vi "AUTO_HOME.vi"(8 "error in (no error)":errorcluster) -> (0 "error out":errorcluster)   [LabVIEW 2017]
doc: "This vi is for manually turn ON and OFF also monitor Output of PLCS. So this is manual screen."
uses:
  b56ad881-f772-481a-9ad8-33fdffb2c092.vi
  Global/PLC_to_Auto.vi
  <vilib>/Utility/file.llb/Read Delimited Spreadsheet (string).vi
  <vilib>/Utility/file.llb/Write Delimited Spreadsheet (string).vi
panel:
  out "AUTO\nHOME STOP":bool
  in  "SPRING ABORT":bool
  in  "SPRING ACK":bool
  out "PART OK":bool
  out "SYSTEM READY":bool
  out "HAUSING STATUS":bool
  out "MAGNETIC STATUS":bool
  out "CBCT STATUS":bool
  out "PMR STATUS":bool
  out "KINEMATIC STATUS":bool
  out "KITTING ST NG COUNTER":u16 format="NG COUNTER: %.0f"
  out "KITTING ST OK COUNTER":u16 format="OK COUNTER: %.0f"
  out "KITTING ST CYCLE TIME":dbl format="CYCLE TIME : %.1f SEC"
  out "CYCLE STATUS 10":bool
  out "CYCLE STATUS 8":bool
  out "CYCLE STATUS 4":bool
  out "CYCLE STATUS 7":bool
  out "CYCLE STATUS 3":bool
  out "CYCLE STATUS 6":bool
  out "CYCLE STATUS 2":bool
  out "CYCLE STATUS 5":bool
  out "CYCLE STATUS 1":bool
  out "CYCLE TIME IN SEC":T1 {"CYCLE TIME 10" format="%.1f"; "CYCLE TIME 8" format="%.1f"; "CYCLE TIME 4" format="%.1f"; "CYCLE TIME 7" format="%.1f"; "CYCLE TIME 3" format="%.1f"; "CYCLE TIME 6" format="%.1f"; "CYCLE TIME 2" format="%.1f"; "CYCLE TIME 5" format="%.1f"; "CYCLE TIME 1" format="%.1f"}
  out "BOOLEAN 2":bool
  out "Plan Selected:":string
  out "USER:-":string
  out "ALARM Indicator":string
  out "DATE/TIME":string
  in  "Back":bool
  # "AUTO HOME"
  # "7.NEUTRAL\n2B ASSEMBLY"
  # "4.NEUTRAL\nIA ASSEMBLY"
  # "6.NEUTRAL\n2A ASSEMBLY"
  # "5.NEUTRAL\nIB ASSEMBLY"
  # "3.PHASE SIDE\nII ASSEMBLY"
  # "10.FINAL\nVISION SYSTEM"
  # "8.NEUTRAL\n2C ASSEMBLY"
  # "2.PHASE SIDE\nI ASSEMBLY"
  # "1.KITTING \nSTATION"
  # "CYCLE TIME IN SEC"
  # "OK COUNTER"
  # "NG COUNTER"
  # "CYCLE STATUS"
  # "ALARM:-"
  # "STATUS OF\n KITTING STATION"
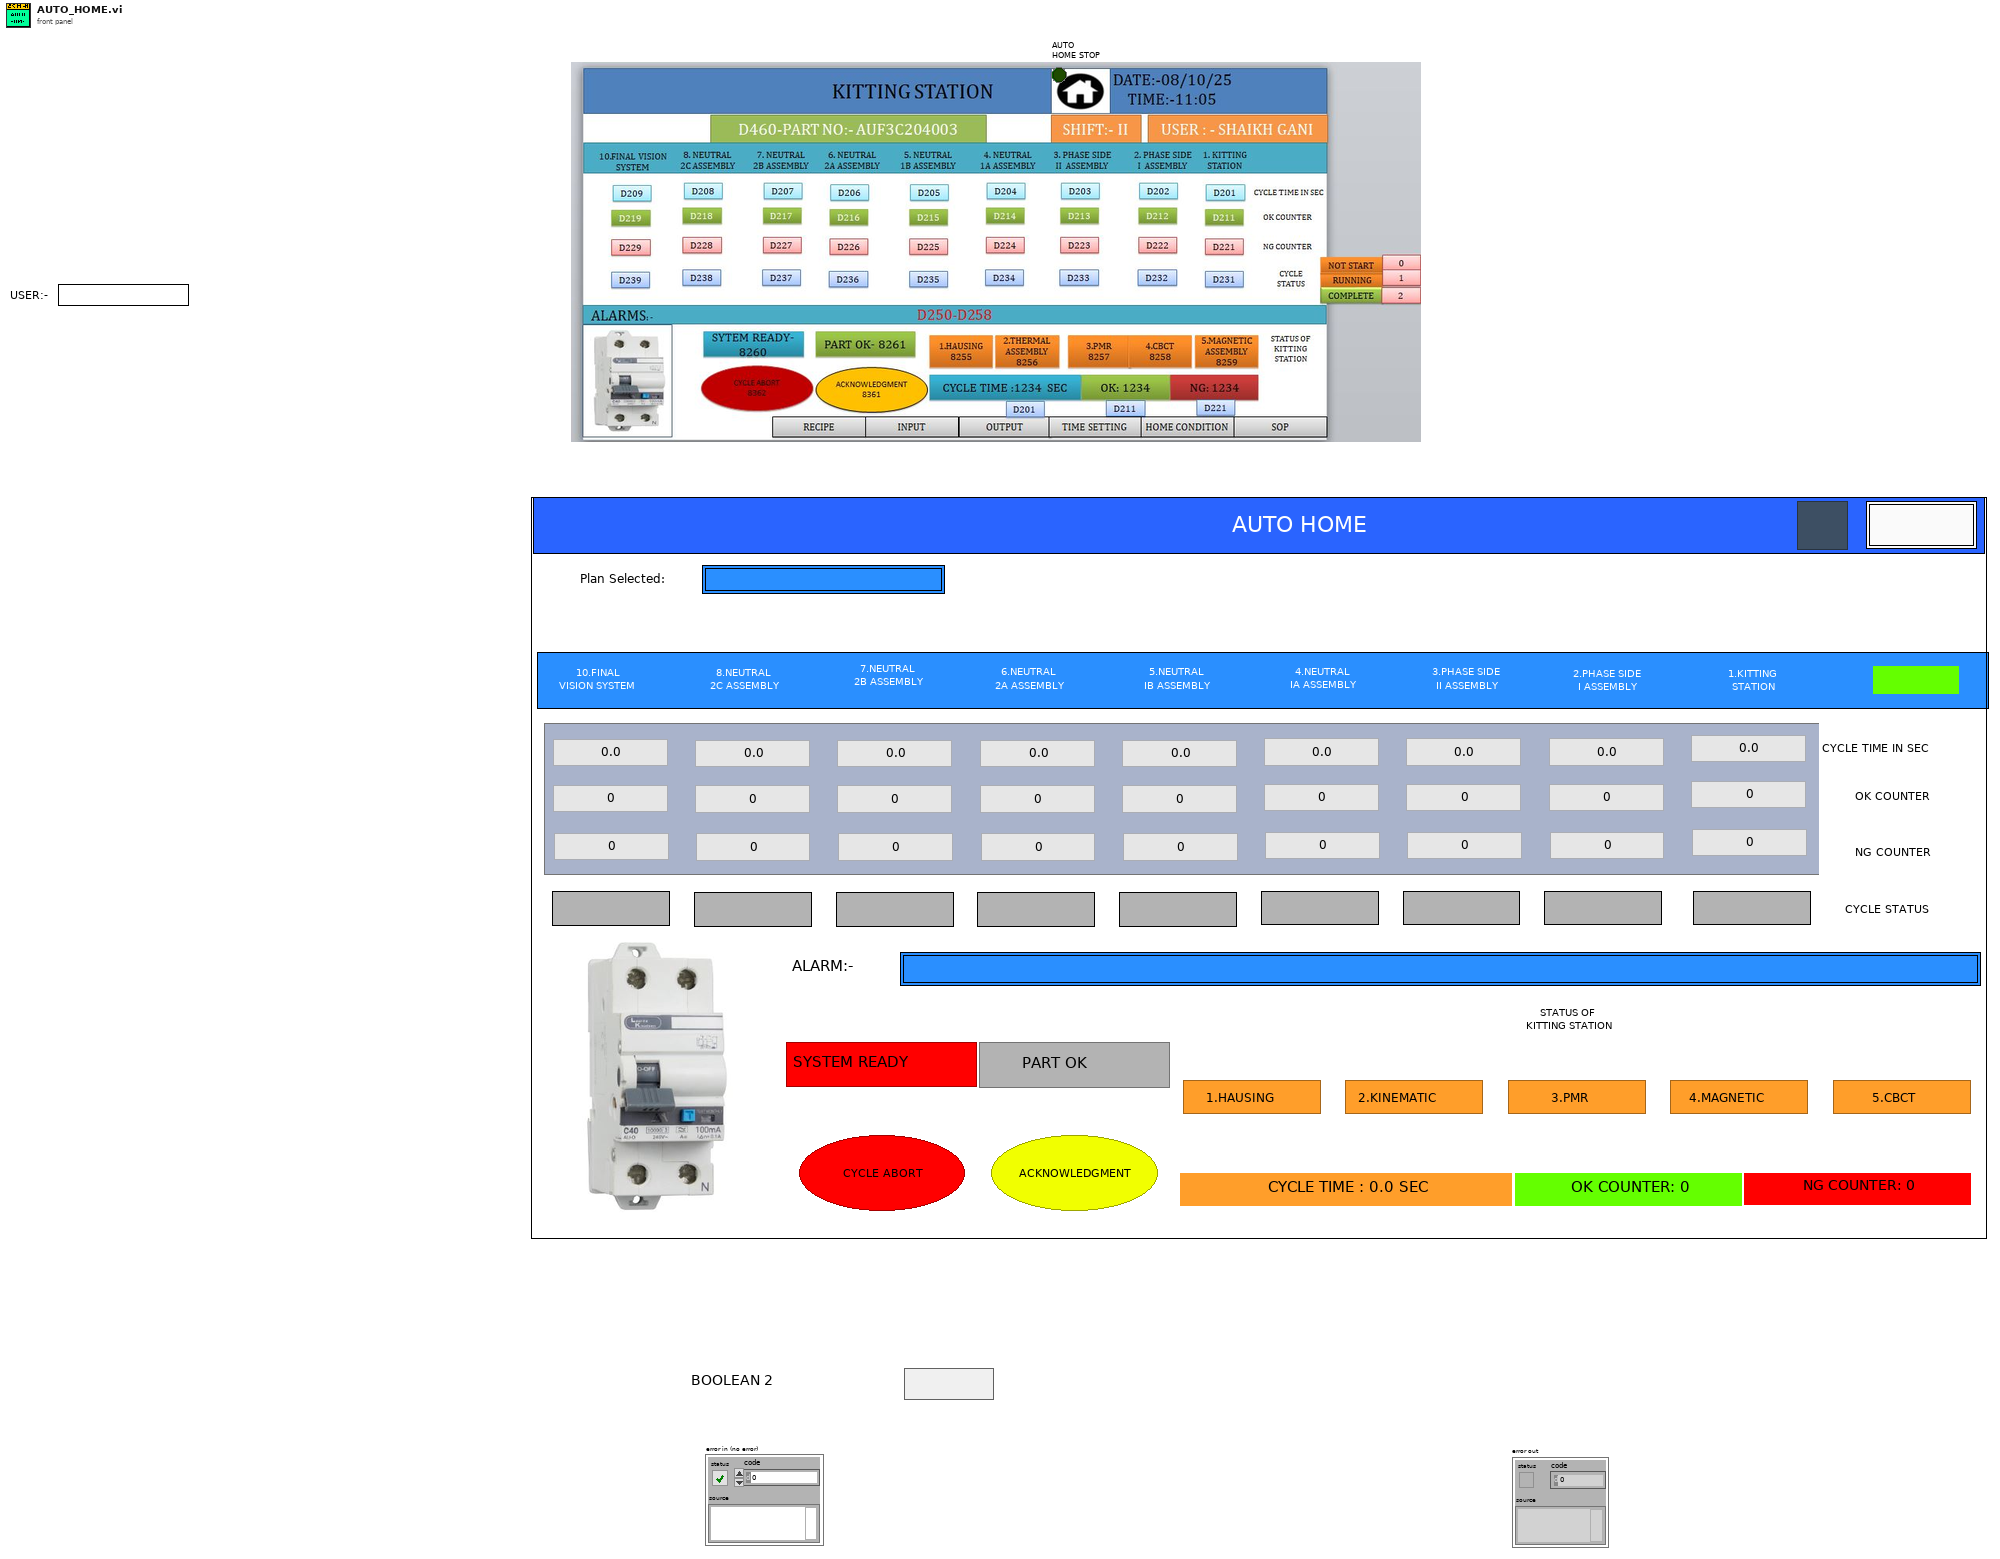
[diagram p1: front panel]
types:
  T1 = cluster{"CYCLE TIME 1":dbl, "CYCLE TIME 2":dbl, "CYCLE TIME 3":dbl, "CYCLE TIME 4":dbl, "CYCLE TIME 5":dbl, "CYCLE TIME 6":dbl, "CYCLE TIME 7":dbl, "CYCLE TIME 8":dbl, "CYCLE TIME 10":dbl, "CYCLE TIME 9":u16, "CYCLE TIME 12":u16, "CYCLE TIME 14":u16, "CYCLE TIME 16":u16, "CYCLE TIME 11":u16, "CYCLE TIME 13":u16, "CYCLE TIME 15":u16, "CYCLE TIME 17":u16, "CYCLE TIME 18":u16, "CYCLE TIME 19":u16, "CYCLE TIME 21":u16, "CYCLE TIME 23":u16, "CYCLE TIME 25":u16, "CYCLE TIME 20":u16, "CYCLE TIME 22":u16, "CYCLE TIME 24":u16, "CYCLE TIME 26":u16, "CYCLE TIME 27":u16}
  T2 = enum32{"invalid app kind", "Development System", "Run Time System", "Student Edition", "Embedded LabVIEW", "Evaluation", "Custom"}
  T3 = cluster{"[0]":dbl, "[1]":dbl, "[2]":dbl, "[3]":dbl, "[4]":dbl, "[5]":dbl, "[6]":dbl, "[7]":dbl, "[8]":dbl, "[9]":dbl, "[10]":dbl, "[11]":dbl, "[12]":dbl, "[13]":dbl, "[14]":dbl, "[15]":dbl, "[16]":dbl, "[17]":dbl, "[18]":dbl, "[19]":dbl, "[20]":dbl, "[21]":dbl, "[22]":dbl, "[23]":dbl, "[24]":dbl, "[25]":dbl, "[26]":dbl}
  T4 = enum32{"Invalid", "Standard", "Closed", "Hidden", "Minimized", "Maximized"}
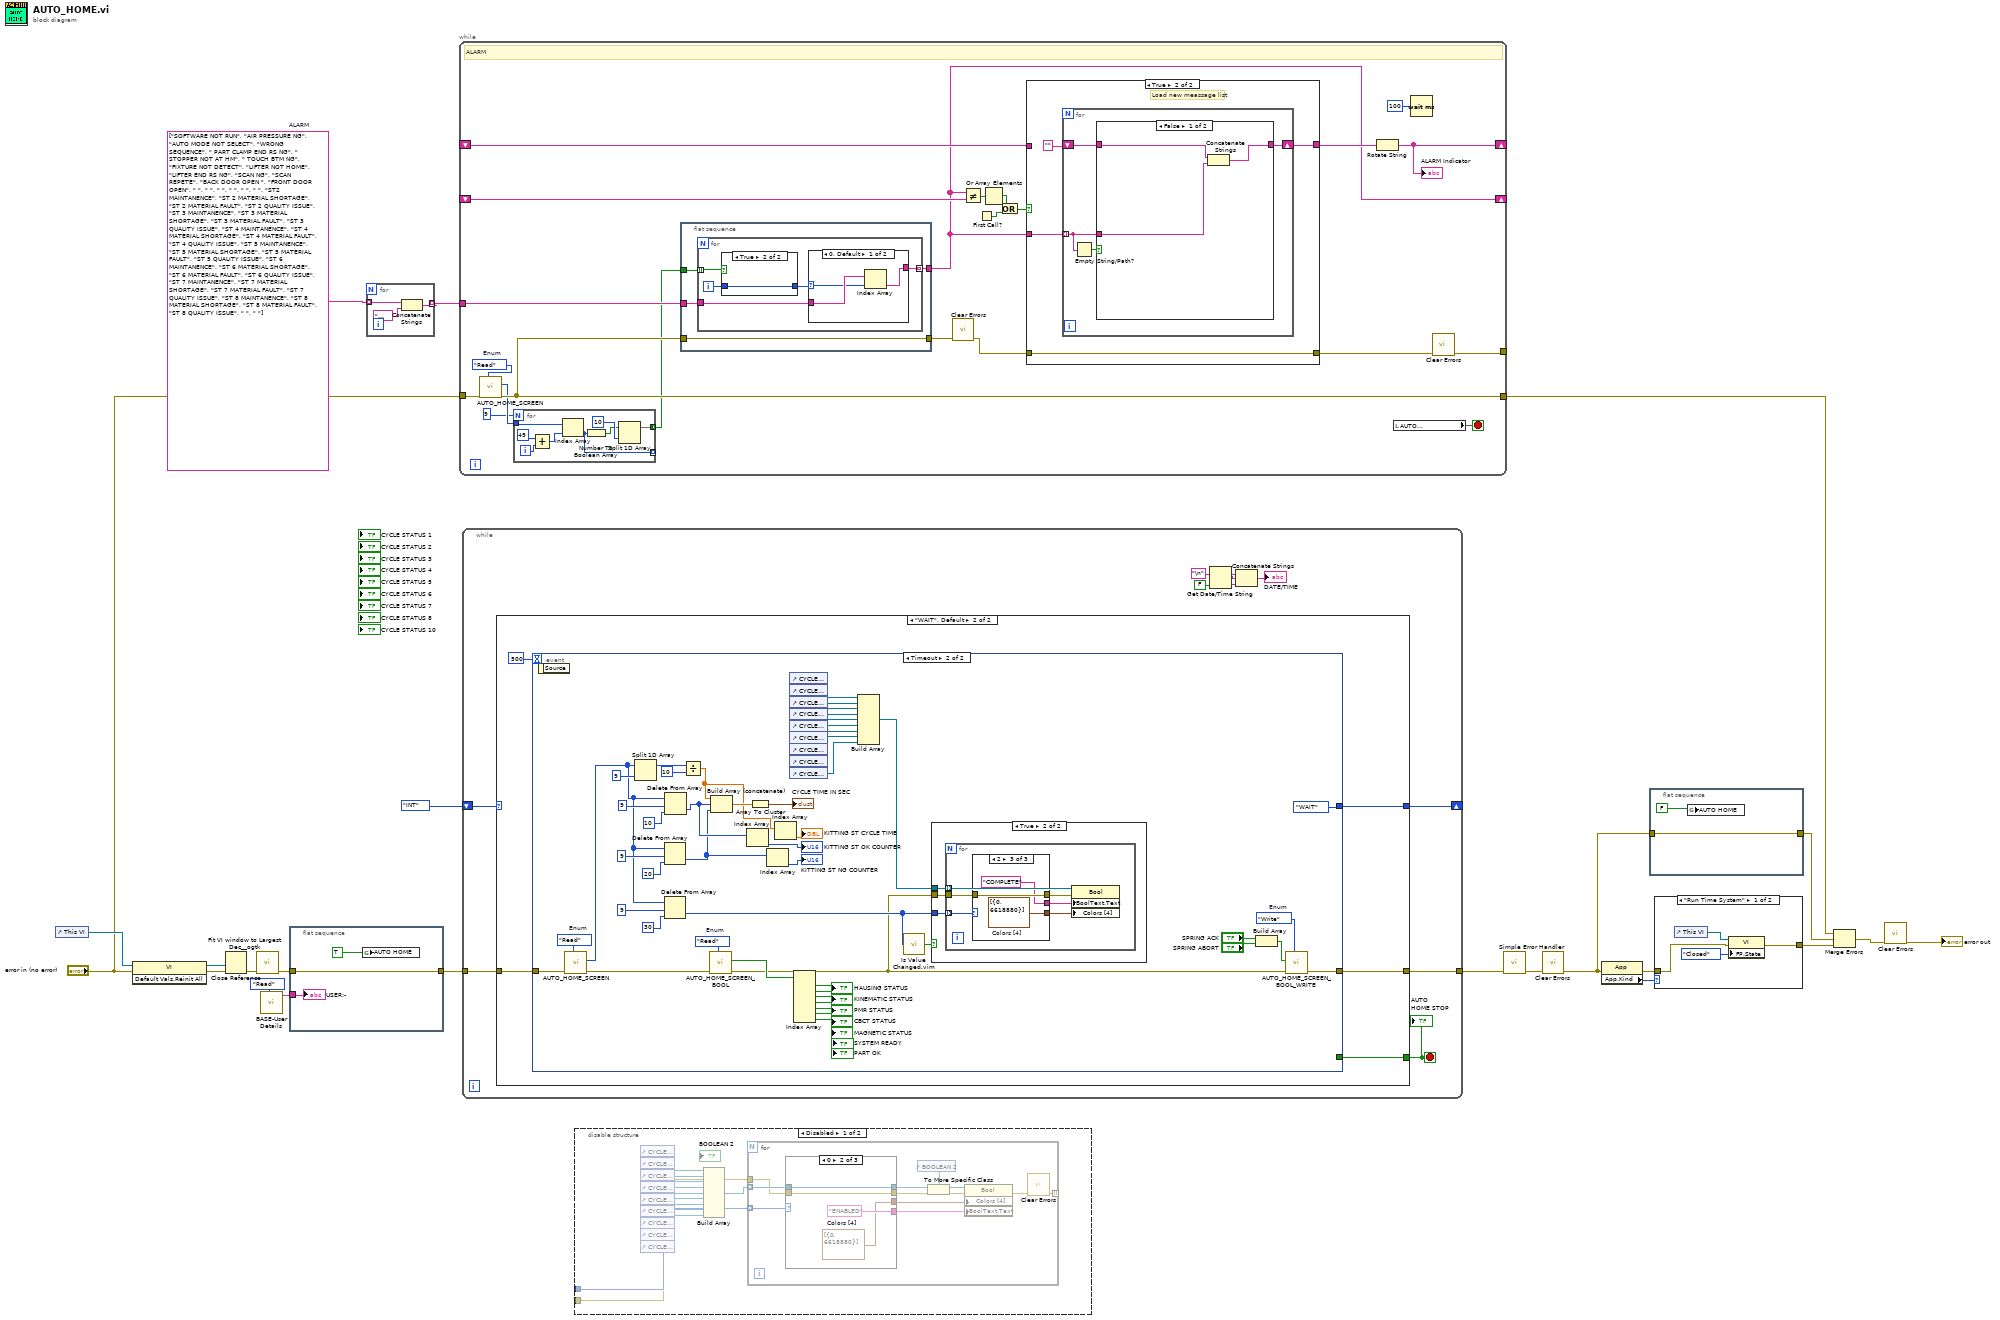
[diagram p0: block diagram]
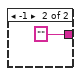
[diagram p2: hidden frame]
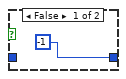
[diagram p3: hidden frame]
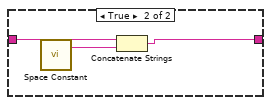
[diagram p5: hidden frame]
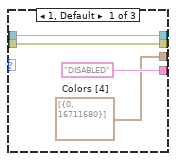
[diagram p6: hidden frame]
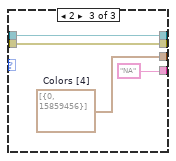
[diagram p7: hidden frame]
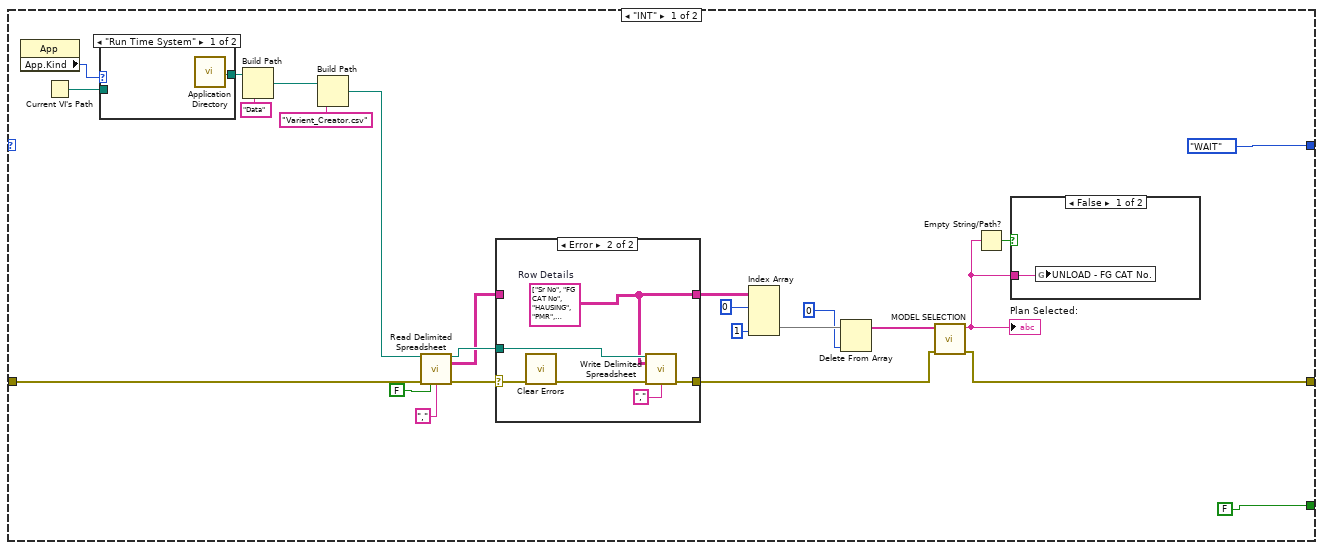
[diagram p10: hidden frame]
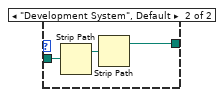
[diagram p12: hidden frame]
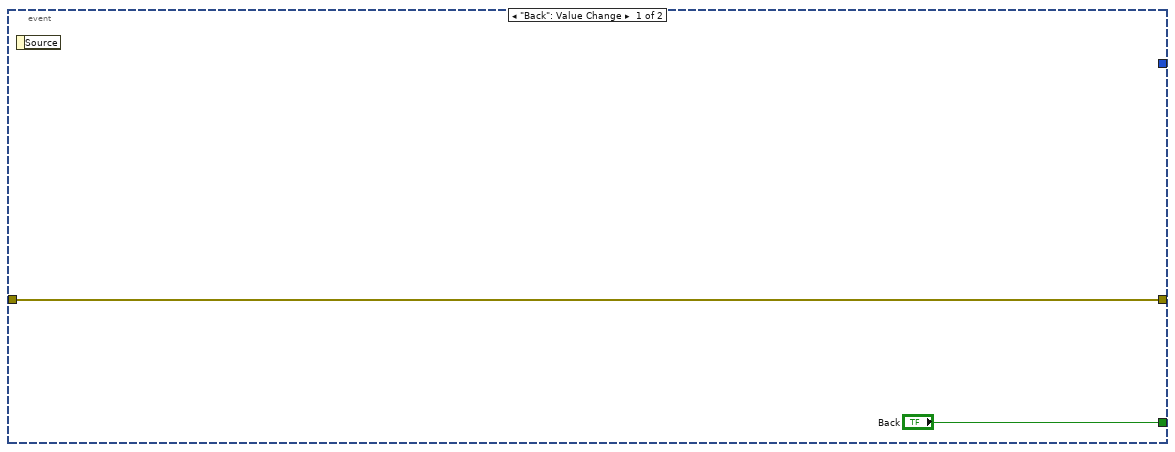
[diagram p14: hidden frame]
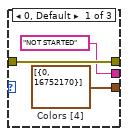
[diagram p16: hidden frame]
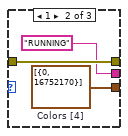
[diagram p17: hidden frame]
diagram:
  w1 = string[] ["SOFTWARE NOT RUN", "AIR PRESSURE NG", "AUTO MODE NOT SELECT", "WRONG SEQUENCE", " PART CLAMP END RS NG", " STOPPER NOT AT HM", " TOUCH BTM NG", "FIXTURE NOT DETECT", "LIFTER NOT HOME", "LIFTER END RS NG", "SCAN NG", "SCAN  REPETE", "BACK DOOR OPEN ", "FRONT DOOR OPEN", " ", " ", " ", " ", " ", " ", "ST2 MAINTANENCE", "ST 2 MATERIAL SHORTAGE", "ST 2 MATERIAL FAULT", "ST 2 QUALITY ISSUE", "ST 3 MAINTANENCE", "ST 3 MATERIAL SHORTAGE", "ST 3 MATERIAL FAULT", "ST 3 QUALITY ISSUE", "ST 4 MAINTANENCE", "ST 4 MATERIAL SHORTAGE", "ST 4 MATERIAL FAULT", "ST 4 QUALITY ISSUE", "ST 5 MAINTANENCE", "ST 5 MATERIAL SHORTAGE", "ST 5 MATERIAL FAULT", "ST 5 QUALITY ISSUE", "ST 6 MAINTANENCE", "ST 6 MATERIAL SHORTAGE", "ST 6 MATERIAL FAULT", "ST 6 QUALITY ISSUE", "ST 7 MAINTANENCE", "ST 7 MATERIAL SHORTAGE", "ST 7 MATERIAL FAULT", "ST 7 QUALITY ISSUE", "ST 8 MAINTANENCE", "ST 8 MATERIAL SHORTAGE", "ST 8 MATERIAL FAULT", "ST 8 QUALITY ISSUE", " ", " "]  # ALARM
  n1 = control-ref of="This VI"() -> (w18:refnum<vi>)
  n2 = invoke class="VI" method="Default Vals.Reinit All"(reference=w18, error in="error in (no error)") -> (reference out=w17:refnum<vi>, error out=w16:errorcluster)  [unwired: 1 in, 1 out]
  n3 = Close Reference(reference=w17, error in (no error)=w16) -> (error out=w15:errorcluster)
  n4 = call <userlib>:"Fit VI window to Largest Dec__ogtk.vi"("error in (no error)"=w15) -> ("error out"=w14:errorcluster)  [unwired: 5 in, 1 out]
  n5 = call "BASE-User Details.vi"("Enum"=enum16{"Read", "Write"}."Read") -> ("User Name Out"=w6:string)  [unwired: 9 in, 1 out]
  n6 = flat-sequence {
    tunnel: w14 -> [w25]
    tunnel: [w25] -> w10
    tunnel: w6 -> [w23]
    frame #0 {
      n7 = global write "PLC_to_Auto.vi" "AUTO HOME"(TRUE) -> ()
      "USER:-" <- w23
    }
  }
  n8 = for {
    tunnel: w1 -> [w28] mode=indexing
    tunnel: [w26] -> w4 mode=indexing
    n9 = Concatenate Strings(w28, "          ") -> (w26:string)
  }
  n10 = while {
    tunnel: "error in (no error)" -> [w34]
    tunnel: [w39] -> _
    tunnel: w4 -> [w37]
    shift-right: [w35] -> _
    shift-left: _ -> [w46]
    shift-right: [w45] -> _
    shift-left: _ -> [w47]
    tunnel: [w33] -> w2
    stop <- w36 stop-if-true
    w32 = enum16{"Read", "Write"}."Read"  # Enum
    # "ALARM"
    n11 = call "AUTO_HOME_SCREEN.vi"("Enum"=w32, "error in (no error)"=w34) -> ("error out"=w33:errorcluster, "Array 2"=w31:u16[])  [unwired: 8 in]
    n12 = for {
      N: 9 -> [_]
      tunnel: w31 -> [w58]
      tunnel: [w52] -> w29 mode=concatenating
      tunnel: [w51] -> _ mode=indexing
      i -> [w56]
      n13 = Add(x=49, y=w56) -> (x+y=w55:i32)
      n14 = Index Array(array=w58, index=w55) -> (element=w51:u16)
      n15 = Number To Boolean Array(number=w51) -> (Boolean array=w53:bool[])
      n16 = Split 1D Array(array=w53, index=10) -> (first subarray=w52:bool[])  [unwired: 1 out]
    }
    n17 = flat-sequence {
      tunnel: [w60] -> w41
      tunnel: [w62] -> w45
      tunnel: w37 -> [w61]
      tunnel: w33 -> [w60]
      tunnel: w29 -> [w59]
      frame #0 {
        n18 = for {
          tunnel: w59 -> [w67] mode=indexing
          tunnel: [w63] -> w62 mode=indexing
          tunnel: w61 -> [w65]
          i -> [w66]
          n19 = case shown="True" w67 {
            tunnel: w66 -> [_ w73]
            tunnel: [-1 w73] -> w64
            frame False {
            }
            frame True {
            }
          }
          n20 = case shown="0, Default" w64 {
            selector: w64 -> [w69 _]
            tunnel: w65 -> [w70 _]
            tunnel: [w68 ""] -> w63
            frame 0, Default {
              n21 = Index Array(array=w70, index=w69) -> (element=w68:string)
            }
            frame -1 {
            }
          }
        }
      }
    }
    n22 = call <vilib>:"Clear Errors.vi"("error in (no error)"=w41) -> ("error out"=w40:errorcluster)  [unwired: 5 in, 1 out]
    n23 = Not Equal?(x=w45, y=w47) -> (x != y?=w49:bool[])
    n24 = First Call?() -> (First Call?: T/F=w44:bool)
    n25 = Or Array Elements(Boolean array=w49) -> (logical OR=w43:bool)
    n26 = Or(x=w43, y=w44) -> (x .or. y?=w42:bool)
    n27 = case shown="True" w42 {
      tunnel: [w75 w77] -> w48
      tunnel: w46 -> [w75 _]
      tunnel: w45 -> [_ w78]
      tunnel: w40 -> [w74 w76]
      tunnel: [w74 w76] -> w38
      frame False {
      }
      frame True {
        # "Load new meassage list"
        n28 = for {
          tunnel: w78 -> [w81] mode=indexing
          shift-right: [w83] -> w77
          shift-left: "" -> [w82]
          n29 = Empty String/Path?(string/path=w81) -> (empty?=w80:bool)
          n30 = case shown="False" w80 {
            tunnel: [w86 w89] -> w83
            tunnel: w82 -> [w85 w88]
            tunnel: w81 -> [w84 _]
            frame False {
              n31 = Concatenate Strings(w85, w84) -> (w86:string)
            }
            frame True {
              n32 = call <vilib>:"Space Constant.vi"() -> ("String"=w87:string)
              n33 = Concatenate Strings(w88, w87) -> (w89:string)
            }
          }
        }
      }
    }
    n34 = Rotate String(1:w48) -> (0:w35:string)
    "ALARM Indicator" <- w35
    n35 = local read "AUTO\nHOME STOP"() -> (w36:bool)
    n36 = Wait (ms)(milliseconds to wait=u32 100) -> ()  [unwired: 1 out]
    n37 = call <vilib>:"Clear Errors.vi"("error in (no error)"=w38) -> ("error out"=w39:errorcluster)  [unwired: 5 in, 1 out]
  }
  n38 = while {
    tunnel: w10 -> [w99]
    tunnel: [w98] -> w21
    shift-right: [w95] -> _
    shift-left: enum16{"INT", "WAIT"}."INT" -> [w96]
    stop <- w97 stop-if-true
    n39 = case shown="\"WAIT\", Default" w96 {
      tunnel: w99 -> [w116 w142]
      tunnel: [w106 w141] -> w98
      tunnel: [FALSE w140] -> w97
      tunnel: [enum16{"INT", "WAIT"}."WAIT" w138] -> w95
      frame "INT" {
        n40 = property class="App"() -> ("App.Kind"=w114:T2)  [unwired: 2 in, 2 out]
        n41 = Current VI's Path() -> (path=w115:path)
        n42 = case shown="\"Run Time System\"" w114 {
          tunnel: w115 -> [_ w128]
          tunnel: [w126 w127] -> w112
          frame "Run Time System" {
            n43 = call <vilib>:"Application Directory.vi"() -> ("Application Directory"=w126:path)
          }
          frame "Development System", Default {
            n44 = Strip Path(path=w128) -> (stripped path=w129:path)  [unwired: 1 out]
            n45 = Strip Path(path=w129) -> (stripped path=w127:path)  [unwired: 1 out]
          }
        }
        n46 = Build Path(base path=w112, name or relative path="Data") -> (appended path=w110:path)
        n47 = Build Path(base path=w110, name or relative path="Varient_Creator.csv") -> (appended path=w109:path)
        n48 = call-poly <vilib>:"Read Delimited Spreadsheet.vi"("file path (dialog if empty)"=w109, "error in (no error)"=w116, "transpose? (F)"=FALSE, "delimiter (\\t)"=",") -> ("new file path (Not A Path if cancelled)"=w121:path, "all rows"=w120:string[][], "error out"=w122:errorcluster)  [unwired: 6 in, 3 out]
        n49 = case shown="Error" w122 {
          selector: w122 -> [w131 w137]
          tunnel: [w131 w135] -> w108
          tunnel: w121 -> [_ w134]
          tunnel: [w130 w132] -> w117
          tunnel: w120 -> [w130 _]
          frame No Error {
          }
          frame Error {
            w132 = string[][] [["Sr No", "FG CAT No", "HAUSING", "PMR", "MAGNETIC ASLY", "CBCT GROUP", "KINEMATIC ASLY", "TEST RESISTOR"]]  # Row Details
            n50 = call <vilib>:"Clear Errors.vi"("error in (no error)"=w137) -> ("error out"=w136:errorcluster)  [unwired: 5 in, 1 out]
            n51 = call-poly <vilib>:"Write Delimited Spreadsheet.vi"("file path (dialog if empty)"=w134, "2D data"=w132, "error in (no error)"=w136, "delimiter (\\t)"=",") -> ("error out"=w135:errorcluster)  [unwired: 10 in, 1 out]
          }
        }
        n52 = Index Array(array=w117, index (row) #1=0, index (col) #2=1) -> (element #2=w104:string[])  [unwired: 2 in, 1 out]
        n53 = Delete From Array(array=w104, index=0) -> (array with subset deleted=w103:string[])  [unwired: 1 in, 1 out]
        n54 = call "MODEL SELECTION.vi"("error in (no error)"=w108, "Plan List"=w103) -> ("error out 2"=w106:errorcluster, "Plan Selected"=w100:string)  [unwired: 7 in, 1 out]
        "Plan Selected:" <- w100
        n55 = Empty String/Path?(string/path=w100) -> (empty?=w101:bool)
        n56 = case shown="False" w101 {
          tunnel: w100 -> [w125 _]
          frame False {
            n57 = global write "PLC_to_Auto.vi" "UNLOAD - FG CAT No."(w125) -> ()
          }
          frame True {
          }
        }
      }
      frame "WAIT", Default {
        n58 = event shown="[1] Timeout" {
          selector: _ -> [_ _]
          dyn-events: _ -> [_ _]
          timeout: 500 -> [_ _]
          tunnel: w142 -> [w143 w191]
          tunnel: [w143 w146] -> w141
          tunnel: ["Back" _] -> w140
          tunnel: [_ enum16{"INT", "WAIT"}."WAIT"] -> w138
          event "Back": Value Change {
            n59 = event-data() -> ()  [unwired: 1 in, 1 out]
          }
          event Timeout {
            w145 = enum16{"Read", "Write"}."Write"  # Enum
            w151 = enum16{"Read", "Write"}."Read"  # Enum
            w192 = enum16{"Read", "Write"}."Read"  # Enum
            n60 = event-data() -> ()  [unwired: 1 in, 1 out]
            n61 = call "AUTO_HOME_SCREEN.vi"("Enum"=w192, "error in (no error)"=w191) -> ("error out"=w152:errorcluster, "Array 2"=w179:u16[])  [unwired: 8 in]
            n62 = Split 1D Array(array=w179, index=9) -> (first subarray=w183:u16[])  [unwired: 1 out]
            n63 = Delete From Array(array=w179, length=9 ("index"), index=20) -> (deleted portion=w161:u16[])  [unwired: 1 out]
            n64 = Delete From Array(array=w179, length=9 ("index"), index=30) -> (deleted portion=w167:u16[])  [unwired: 1 out]
            n65 = Delete From Array(array=w179, length=9 ("index"), index=10) -> (deleted portion=w162:u16[])  [unwired: 1 out]
            n66 = Divide(x=w183, y=10 ("index")) -> (x/y=w163:dbl[])
            n67 = call "AUTO_HOME_SCREEN_BOOL.vi"("Enum"=w151, "error in (no error)"=w152) -> ("error out"=w147:errorcluster, "Array 2"=w153:bool[])  [unwired: 8 in]
            n68 = Build Array (concatenate)(w163, w162, w161) -> (w186:dbl[])
            n69 = Index Array(array=w162) -> (element=→"KITTING ST OK COUNTER":u16)  [unwired: 1 in]
            n70 = Array To Cluster(array=w186) -> (cluster=→"CYCLE TIME IN SEC":T3)
            n71 = Index Array(array=w161) -> (element=→"KITTING ST NG COUNTER":u16)  [unwired: 1 in]
            n72 = Index Array(array=w163) -> (element=→"KITTING ST CYCLE TIME":dbl)  [unwired: 1 in]
            n73 = control-ref of="CYCLE STATUS 1"() -> (w178:refnum<vi>)
            n74 = control-ref of="CYCLE STATUS 2"() -> (w177:refnum<vi>)
            n75 = control-ref of="CYCLE STATUS 3"() -> (w176:refnum<vi>)
            n76 = control-ref of="CYCLE STATUS 4"() -> (w175:refnum<vi>)
            n77 = control-ref of="CYCLE STATUS 5"() -> (w174:refnum<vi>)
            n78 = control-ref of="CYCLE STATUS 6"() -> (w173:refnum<vi>)
            n79 = control-ref of="CYCLE STATUS 7"() -> (w172:refnum<vi>)
            n80 = control-ref of="CYCLE STATUS 8"() -> (w171:refnum<vi>)
            n81 = control-ref of="CYCLE STATUS 10"() -> (w170:refnum<vi>)
            n82 = Index Array(array=w153) -> (element #1=→"HAUSING STATUS":bool, element #2=→"KINEMATIC STATUS":bool, element #3=→"PMR STATUS":bool, element #4=→"CBCT STATUS":bool, element #5=→"MAGNETIC STATUS":bool, element #6=→"SYSTEM READY":bool, element #7=→"PART OK":bool)  [unwired: 7 in]
            n83 = Build Array(w178, w177, w176, w175, w174, w173, w172, w171, w170) -> (w169:refnum<vi>[])
            n84 = call "Is Value Changed.vim"("value"=w167) -> ("changed or first call?"=w168:bool)
            n85 = case shown="True" w168 {
              tunnel: w169 -> [_ w196]
              tunnel: w167 -> [_ w195]
              tunnel: w147 -> [_ w194]
              frame False {
              }
              frame True {
                n86 = for {
                  tunnel: w196 -> [w202] mode=indexing
                  tunnel: w195 -> [w199] mode=indexing
                  tunnel: w194 -> [w201]
                  n87 = case shown="2" w199 {
                    tunnel: w201 -> [w205 w208 w211]
                    tunnel: [w205 w208 w211] -> w200
                    tunnel: [w204 w207 w210] -> w198
                    tunnel: ["NOT STARTED" "RUNNING" "COMPLETE"] -> w197
                    frame 0, Default {
                      w204 = cluster{u32, u32}[] [{0, 16752170}]  # Colors [4]
                    }
                    frame 1 {
                      w207 = cluster{u32, u32}[] [{0, 16752170}]  # Colors [4]
                    }
                    frame 2 {
                      w210 = cluster{u32, u32}[] [{0, 6618880}]  # Colors [4]
                    }
                  }
                  n88 = property class="Bool"(reference=w202, error in=w200, "BoolText.Text"=w197, "Colors [4]"=w198) -> ()  [unwired: 2 out]
                }
              }
            }
            n89 = Build Array("SPRING ACK", "SPRING ABORT") -> (w148:bool[])
            n90 = call "AUTO_HOME_SCREEN_BOOL_WRITE.vi"("Enum"=w145, "error in (no error)"=w147, "Array"=w148) -> ("error out"=w146:errorcluster)  [unwired: 7 in, 1 out]
          }
        }
      }
    }
    "AUTO\nHOME STOP" <- w97
    n91 = Get Date/Time String(want seconds? (F)=FALSE) -> (date string=w94:string, time string=w93:string)  [unwired: 2 in]
    n92 = Concatenate Strings(w94, "\n", w93) -> (→"DATE/TIME":string)
  }
  n93 = disable-structure shown="Disabled" {
    disable-tunnel: _ -> [w213 _]
    disable-tunnel: _ -> [w212 _]
    frame Disabled {
      n94 = control-ref of="CYCLE TIME 1"() -> (w223:refnum<vi>)
      n95 = control-ref of="CYCLE TIME 2"() -> (w222:refnum<vi>)
      n96 = control-ref of="CYCLE TIME 3"() -> (w221:refnum<vi>)
      n97 = control-ref of="CYCLE TIME 4"() -> (w220:refnum<vi>)
      n98 = control-ref of="CYCLE TIME 5"() -> (w219:refnum<vi>)
      n99 = control-ref of="CYCLE TIME 6"() -> (w218:refnum<vi>)
      n100 = control-ref of="CYCLE TIME 7"() -> (w217:refnum<vi>)
      n101 = control-ref of="CYCLE TIME 8"() -> (w216:refnum<vi>)
      n102 = control-ref of="CYCLE TIME 10"() -> (w215:refnum<vi>)
      n103 = Build Array(w223, w222, w221, w220, w219, w218, w217, w216, w215) -> (w214:refnum<vi>[])
      n104 = for {
        tunnel: w213 -> [w235] mode=indexing
        tunnel: w214 -> [w234] mode=indexing
        tunnel: w212 -> [w227]
        tunnel: [w224] -> _ mode=indexing
        n105 = case shown="0" w235 {
          tunnel: w234 -> [w239 w242 w246]
          tunnel: [w239 w242 w246] -> w233
          tunnel: ["DISABLED" "ENABLED" "NA"] -> w230
          tunnel: [w237 w241 w245] -> w229
          tunnel: w227 -> [w236 w240 w244]
          tunnel: [w236 w240 w244] -> w226
          frame 1, Default {
            w237 = cluster{u32, u32}[] [{0, 16711680}]  # Colors [4]
          }
          frame 0 {
            w241 = cluster{u32, u32}[] [{0, 6618880}]  # Colors [4]
          }
          frame 2 {
            w245 = cluster{u32, u32}[] [{0, 15859456}]  # Colors [4]
          }
        }
        n106 = control-ref of="BOOLEAN 2"() -> (w231:refnum<vi>)
        n107 = To More Specific Class(target class=w231, reference=w233, error in=w226) -> (specific class reference=w232:refnum<vi>, error out=w228:errorcluster)
        n108 = property class="Bool"(reference=w232, error in=w228, "Colors [4]"=w229, "BoolText.Text"=w230) -> (error out=w225:errorcluster)  [unwired: 1 out]
        n109 = call <vilib>:"Clear Errors.vi"("error in (no error)"=w225) -> ("error out"=w224:errorcluster)  [unwired: 5 in, 1 out]
      }
    }
    frame Enabled {
    }
  }
  n110 = call <vilib>:"Simple Error Handler.vi"("error in (no error)"=w21) -> ("error out"=w13:errorcluster)  [unwired: 4 in, 4 out]
  n111 = call <vilib>:"Clear Errors.vi"("error in (no error)"=w13) -> ("error out"=w9:errorcluster)  [unwired: 5 in, 1 out]
  n112 = property class="App"(error in=w9) -> (error out=w11:errorcluster, "App.Kind"=w12:T2)  [unwired: 1 in, 1 out]
  n113 = flat-sequence {
    tunnel: w9 -> [w249]
    tunnel: [w249] -> w8
    frame #0 {
      n114 = global write "PLC_to_Auto.vi" "AUTO HOME"(FALSE) -> ()
    }
  }
  n115 = case shown="\"Run Time System\"" w12 {
    tunnel: w11 -> [w251 w254]
    tunnel: [w250 w254] -> w19
    frame "Run Time System" {
      n116 = control-ref of="This VI"() -> (w253:refnum<vi>)
      n117 = property class="VI"(reference=w253, error in=w251, "FP.State"=T4."Closed" ("Front Panel Window:State")) -> (error out=w250:errorcluster)  [unwired: 1 out]
    }
    frame "Development System", Default {
    }
  }
  n118 = Merge Errors(w2, w8, w19) -> (w20:errorcluster)
  n119 = call <vilib>:"Clear Errors.vi"("error in (no error)"=w20) -> ("error out"=→"error out":errorcluster)  [unwired: 5 in, 1 out]
